vi "UDP__TransmitData.vi"(4 "Remote Port":u16=33332, 6 "Remote MAC Address (hex)":string="\u0000\u0000\u0000\u0000\u0000\u0000", 7 "Local Port":u16, 8 "error in":errorcluster, 10 "Parameters":string, 11 "Command":string) -> (0 "error out":errorcluster)   [LabVIEW 2020, in "hse-network.lvlib"]
doc: "____\nHAMPEL SOFTWARE ENGINEERING v3.8.0 (2023-12-18 14:41)"
uses:
  hse-network.lvlib
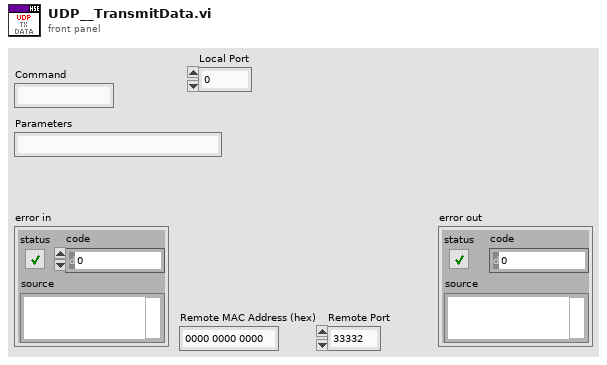
[diagram p1: front panel]
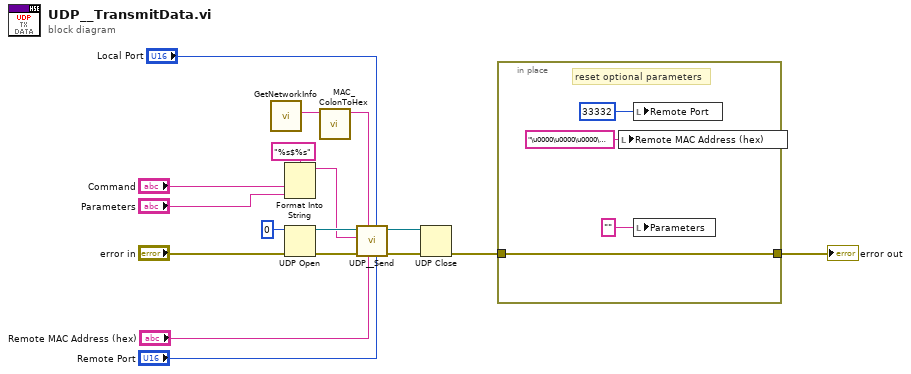
[diagram p0: block diagram]
diagram:
  n1 = call "GetNetworkInfo.vi"() -> ("MAC Address"=w3:string)  [unwired: 9 in, 2 out]
  n2 = Format Into String(format string="%s$%s", "Command", "Parameters") -> (resulting string=w6:string)  [unwired: 2 in, 1 out]
  n3 = UDP Open(8:"error in", 11:u16 0 ("port")) -> (port=w11:refnum<k16>, 0:w8:errorcluster)  [unwired: 4 out]
  n4 = call "MAC_ColonToHex.vi"("MAC Address (colon notation)"=w3) -> ("MAC Address (hex string)"=w1:string)  [unwired: 10 in]
  n5 = call "UDP__Send.vi"("Remote Port"="Remote Port", "Local Port"="Local Port", "Remote MAC Address (hex)"="Remote MAC Address (hex)", "Local MAC Address (hex)"=w1, "error in"=w8, "Command and Data"=w6, "UDP Network Connection in"=w11) -> ("error out"=w9:errorcluster, "UDP Network Connection out"=w10:refnum<k16>)  [unwired: 3 in]
  n6 = UDP Close(connection ID=w10, 8:w9) -> (error out=w13:errorcluster)  [unwired: 1 out]
  n7 = in-place {
    in-place-border: w13 -> [w21]
    in-place-border: [w21] -> w12
    # "reset optional parameters"
    n8 = local write "Remote MAC Address (hex)"("\u0000\u0000\u0000\u0000\u0000\u0000" ("Remote MAC Address")) -> ()
    n9 = local write "Remote Port"(u16 33332 ("Local Port No.")) -> ()
    n10 = local write "Parameters"("" ("Parameters")) -> ()
  }
  "error out" <- w12
